vi "Write Data Server.vi"(8 "error in (no error)":errorcluster, 10 "veristand-grpc_server.lvlib:Data Server.lvclass":refnum<class "Data Server.lvclass">, 11 "veristand in":refnum<class "veristand-grpc.lvclass">) -> (0 "error out":errorcluster, 3 "veristand out":refnum<class "veristand-grpc.lvclass">)   [LabVIEW 2020, in "Veristandgrpc_server.lvlib" / "veristand-grpc.lvclass"]
uses:
  veristand-grpc.lvclass
  Data/Data Server.lvclass
  veristand-grpc.lvclass/veristand-grpc.ctl
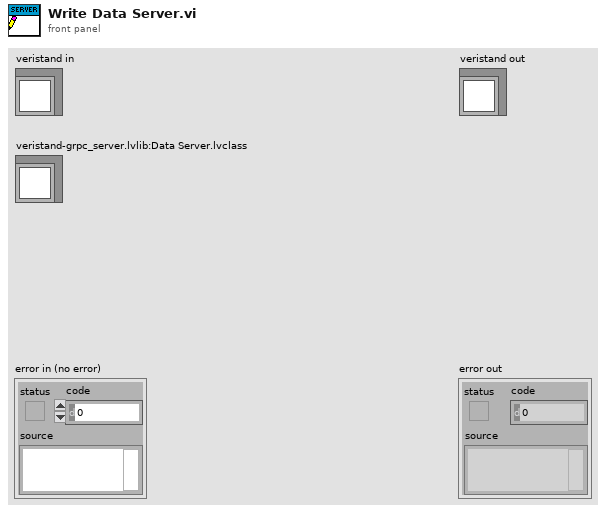
[diagram p1: front panel]
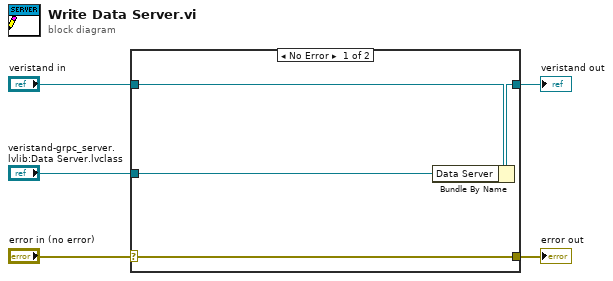
[diagram p0: block diagram]
diagram:
  n1 = case shown="No Error" "error in (no error)" {
    selector: "error in (no error)" -> [w9 w10]
    tunnel: [w9 w10] -> w4
    tunnel: [w7 w11] -> w2
    tunnel: "veristand in" -> [w8 w11]
    tunnel: "veristand-grpc_server.lvlib:Data Server.lvclass" -> [w6 _]
    frame No Error {
      n2 = Bundle By Name(cluster=w8, "Data Server"=w6) -> (w7:refnum<class "veristand-grpc.lvclass">)
    }
    frame Error {
    }
  }
  "error out" <- w4
  "veristand out" <- w2
